vi "Calculate Ouput Level for Digital Audio.vi"(8 "output range (pk-pk)":dbl, 10 "digital output level units":T1, 11 "output level":dbl) -> (1 "amplitude (pk)":dbl, 3 "gain":dbl)   [LabVIEW 2021]
uses:
  controls/digital output level units.ctl
  controls/audio controls.lvlib
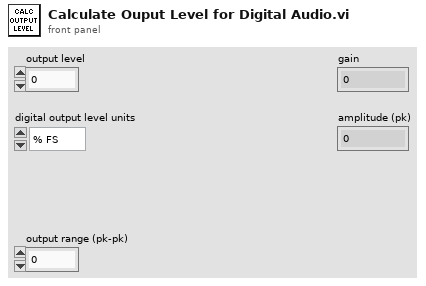
[diagram p1: front panel]
types:
  T1 = typedef "audio controls.lvlib/digital output level units.ctl" = enum32{"% FS", "dBFS"}
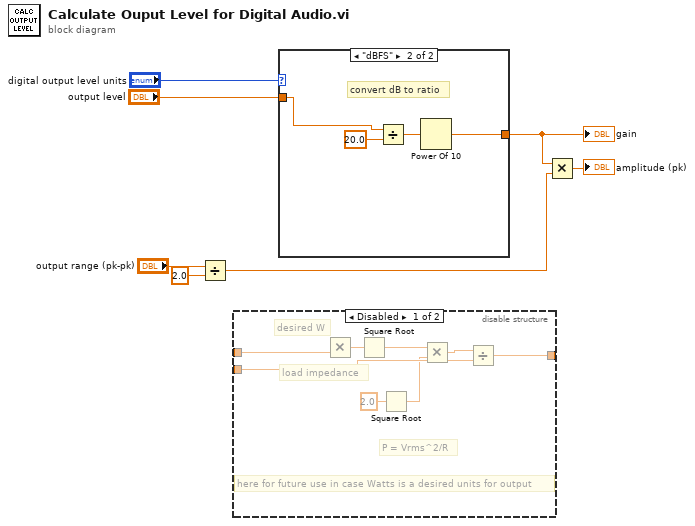
[diagram p0: block diagram]
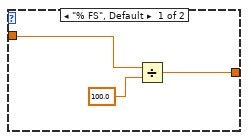
[diagram p3: hidden frame]
diagram:
  n1 = Divide(x="output range (pk-pk)", y=2.0) -> (x/y=w3:dbl)
  n2 = disable-structure shown="Disabled" {
    disable-tunnel: _ -> [w15 _]
    disable-tunnel: [w14 _] -> _
    disable-tunnel: _ -> [w13 _]
    frame Disabled {
      # "here for future use in case Watts is a desired units for output"
      # "desired W"
      # "load impedance"
      # "P = Vrms^2/R"
      n3 = Multiply(y=w13) -> (x=w12:dbl, x*y=w11:dbl)
      n4 = Square Root(x=w11) -> (sqrt(x)=w8:dbl)
      n5 = Square Root(x=2.0) -> (sqrt(x)=w9:dbl)
      n6 = Multiply(x=w8, y=w9) -> (x*y=w10:dbl)
      n7 = Divide(x=w10, y=w15) -> (x/y=w14:dbl)
    }
    frame Enabled {
    }
  }
  n8 = case shown="\"dBFS\"" "digital output level units" {
    tunnel: [w18 w21] -> w5
    tunnel: "output level" -> [w19 w20]
    frame "% FS", Default {
      n9 = Divide(x=w19, y=100.0) -> (x/y=w18:dbl)
    }
    frame "dBFS" {
      # "convert dB to ratio"
      n10 = Divide(x=w20, y=20.0) -> (x/y=w23:dbl)
      n11 = Power Of 10(x=w23) -> (10^x=w21:dbl)
    }
  }
  "gain" <- w5
  n12 = Multiply(x=w5, y=w3) -> (x*y=→"amplitude (pk)":dbl)
